vi "Get Brightness.vi"(8 "error in (no error)":errorcluster caption="错误输入（无错误）", 11 "Color 输入":refnum<class "Color.lvclass"> caption="DNL_LabVIEW Object in") -> (0 "error out":errorcluster caption="错误输出", 2 "GetBrightness":sgl, 3 "Color 输出":refnum<class "Color.lvclass"> caption="DNL_LabVIEW Object out")   [LabVIEW 2012, in "Color.lvclass"]
uses:
  Color.lvclass
  Color.lvclass/Color.ctl
  System.Drawing
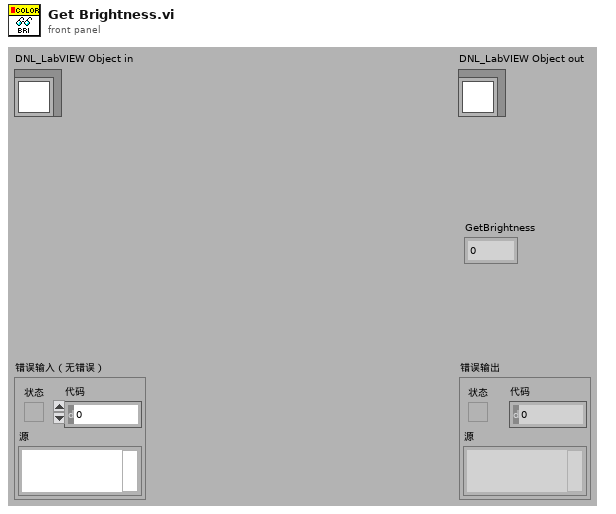
[diagram p1: front panel]
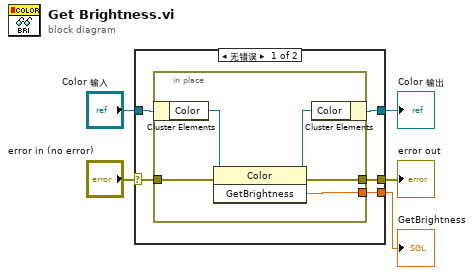
[diagram p0: block diagram]
diagram:
  n1 = case shown="无错误" "error in (no error)" {
    selector: "error in (no error)" -> [w7 w17]
    tunnel: [w6 w17] -> w4
    tunnel: [w9 w16] -> w2
    tunnel: "Color 输入" -> [w10 w16]
    tunnel: [w8 _] -> w1
    frame No Error {
      n2 = in-place {
        in-place-border: [w13] -> w8
        in-place-border: w7 -> [w12]
        in-place-border: [w11] -> w6
        n3 = in-place-cluster #1(w10) -> ("Color"=w15:refnum<k24>)
        n4 = invoke class="Color" method="GetBrightness"(reference=w15, error in=w12) -> (reference out=w14:refnum<k24>, error out=w11:errorcluster, "GetBrightness"=w13:sgl)  [unwired: 1 in]
        n5 = in-place-cluster #1("Color"=w14) -> (w9:refnum<class "Color.lvclass">)
      }
    }
    frame Error {
    }
  }
  "error out" <- w4
  "Color 输出" <- w2
  "GetBrightness" <- w1
